vi "New Queue Mailbox.vi"(5 "Self Alias":string, 7 "Self":refnum<data-value>, 9 "Creator Alias":string, 11 "Creator":refnum<data-value>, 12 "Created":map{string, refnum<data-value>}(c390), 13 "Event":map{string, refnum<data-value>}(c390)) -> (6 "Queue Mailbox":refnum<data-value>, 15 "error out":errorcluster)   [LabVIEW 2021, in "jettl.lvlib"]
uses:
  jettl.lvlib
  Queue Mailbox/Queue Mailbox.lvclass
  Msg Strategy/Msg Strategy.lvclass
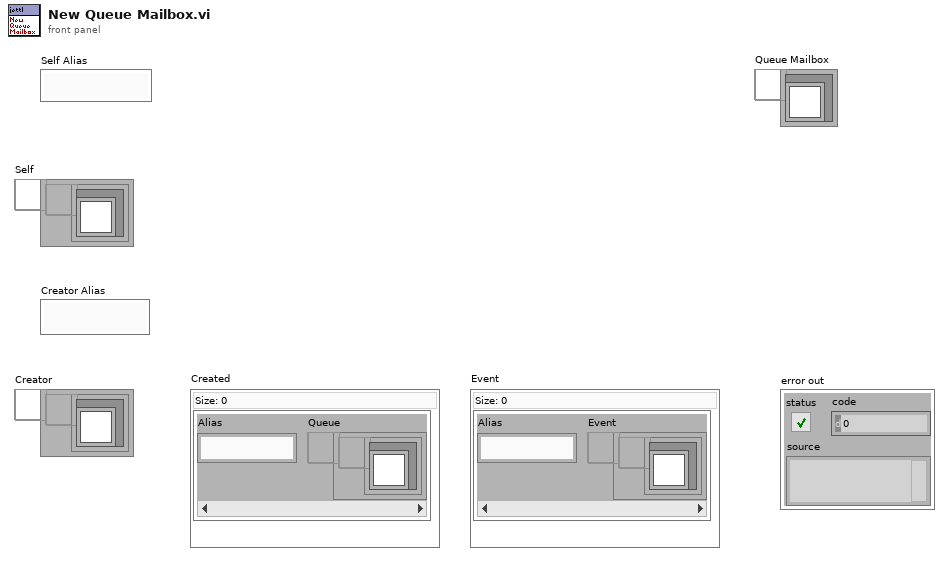
[diagram p1: front panel]
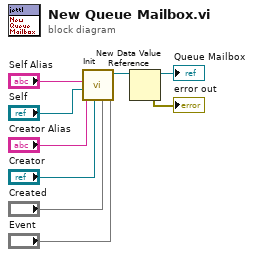
[diagram p0: block diagram]
diagram:
  n1 = call "Init.vi"("Event"="Event", "Created"="Created", "Creator"="Creator", "Creator Alias"="Creator Alias", "Self"="Self", "Self Alias"="Self Alias") -> ("Queue Mailbox out"=w1:refnum<class "Queue Mailbox.lvclass">)  [unwired: 5 in]
  n2 = New Data Value Reference(data value=w1) -> (data value reference=→"Queue Mailbox":refnum<data-value>, error out=→"error out":errorcluster)  [unwired: 1 in]
